vi "oa_Remove Waveform Reference.vi"(0 "resampled signal":cluster{"r0":dbl, "dr":dbl, "Y":dbl[]}={"r0"=0.0, "dr"=1.0, "Y"=[]} {"r0" format="%.2p"; "dr" format="%.2p"; "Y" format="%.2f"}, 5 "baseline in":cluster{"r0":dbl, "dr":dbl, "Y":dbl[]}={"r0"=0.0, "dr"=1.0, "Y"=[]} {"r0" format="%.2p"; "dr" format="%.2p"; "Y" format="%.2f"}, 9 "last index":i32=1, 11 "error out in":errorcluster) -> (4 "compensated signal":cluster{"r0":dbl, "dr":dbl, "Y":dbl[]}={"r0"=0.0, "dr"=1.0, "Y"=[]} {"r0" format="%.2p"; "dr" format="%.2p"; "Y" format="%.2f"}, 10 "last index out":i32=1, 15 "error out":errorcluster)   [LabVIEW 2017, in "SoundVib_RefDataProcess.lvlib"]
uses:
  <vilib>/addons/Sound and Vibration/Order Analysis/Referece Data Processing/SoundVib_RefDataProcess.lvlib
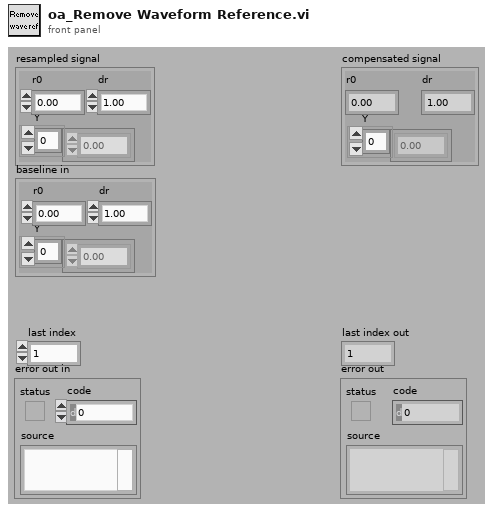
[diagram p1: front panel]
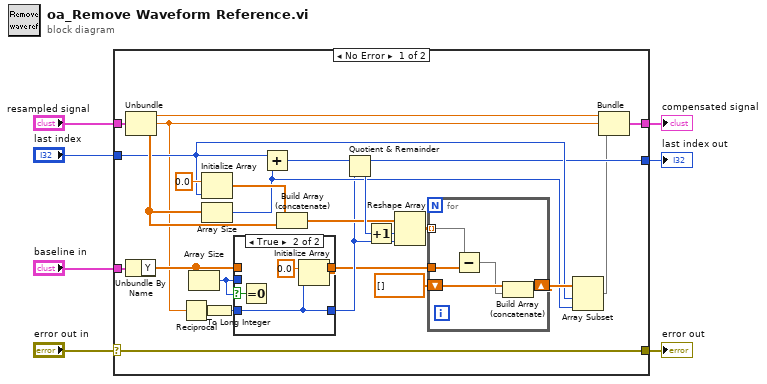
[diagram p0: block diagram]
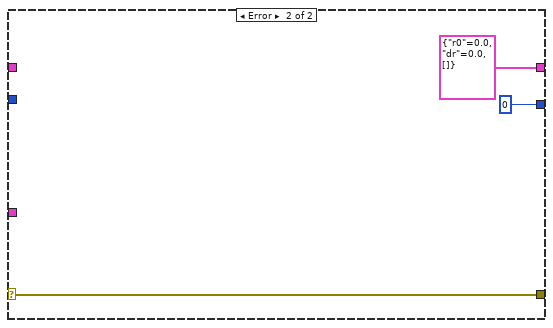
[diagram p3: hidden frame]
diagram:
  n1 = case shown="No Error" "error out in" {
    selector: "error out in" -> [w34 w47]
    tunnel: [w34 w47] -> w6
    tunnel: "resampled signal" -> [w33 _]
    tunnel: "baseline in" -> [w32 _]
    tunnel: "last index" -> [w18 _]
    tunnel: [w17 0] -> w2
    tunnel: [w30 cluster{"r0":dbl, "dr":dbl, dbl[]} {"r0"=0.0, "dr"=0.0, []}] -> w1
    frame No Error {
      n2 = Unbundle(w33) -> ("r0"=w31:dbl, "dr"=w8:dbl, "Y"=w19:dbl[])
      n3 = Unbundle By Name(w32) -> ("Y"=w10:dbl[])
      n4 = Reciprocal(x=w8) -> (1/x=w15:dbl)
      n5 = Array Size(array=w10) -> (size(s)=w13:i32)
      n6 = Initialize Array(0.0 ("element"), w18) -> (w28:dbl[])
      n7 = Array Size(array=w19) -> (size(s)=w20:i32)
      n8 = To Long Integer(number=w15) -> (32bit integer=w12:i32)
      n9 = Equal To 0?(x=w13) -> (x = 0?=w14:bool)
      n10 = case shown="True" w14 {
        tunnel: w13 -> [w36 _]
        tunnel: w12 -> [_ w39]
        tunnel: [w36 w39] -> w11
        tunnel: w10 -> [w35 _]
        tunnel: [w35 w38] -> w9
        frame False {
        }
        frame True {
          n11 = Initialize Array(0.0 ("element"), w39) -> (w38:dbl[])
        }
      }
      n12 = Add(x=w18, y=w20) -> (x+y=w27:i32)
      n13 = Build Array (concatenate)(w28, w19) -> (w25:dbl[])
      n14 = Quotient & Remainder(x=w27, y=w11) -> (x-y*floor(x/y)=w17:i32, floor(x/y)=w26:i32)
      n15 = Increment(x=w26) -> (x+1=w24:i32)
      n16 = Reshape Array(w25, w24, w11) -> (w23:dbl[][])
      n17 = for {
        tunnel: w23 -> [w44] mode=indexing
        tunnel: w9 -> [w43]
        shift-right: [w40] -> w21
        shift-left: dbl[] [] -> [w42]
        n18 = Subtract(x=w44, y=w43) -> (x-y=w41:dbl[])
        n19 = Build Array (concatenate)(w42, w41) -> (w40:dbl[])
      }
      n20 = Array Subset(array=w21, index=w18, length=w20) -> (w16:dbl[])
      n21 = Bundle("r0"=w31, "dr"=w8, w16) -> (w30:cluster{"r0":dbl, "dr":dbl, dbl[]})  [unwired: 1 in]
    }
    frame Error {
    }
  }
  "compensated signal" <- w1
  "error out" <- w6
  "last index out" <- w2
